vi "TCL Select Fragments 1fragNcriteria.vi"(0 "event file":path, 1 "fragment":string, 3 "primary key":string, 4 "criteria":T1(array[cluster]), 5 "error in (no error)":errorcluster) -> (6 "fragments out":string[](array[string]), 7 "matches":string[][](array[string]), 8 "error out":errorcluster)   [LabVIEW 2010]
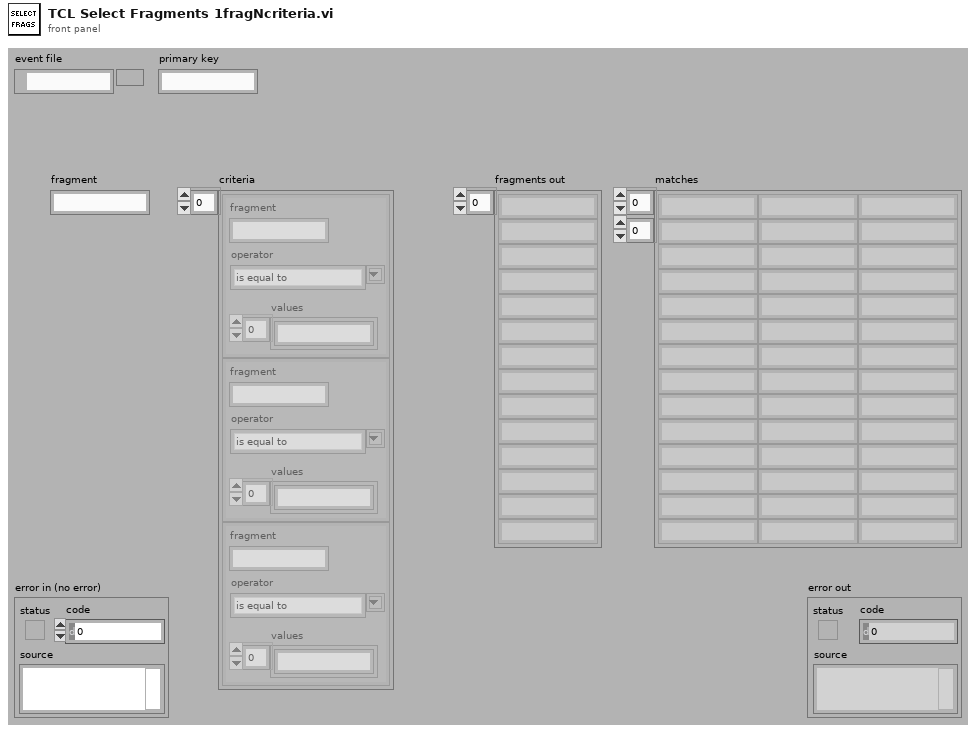
[diagram p1: front panel]
types:
  T1 = cluster{"fragment":string, "values":string[], "operator":string}[]
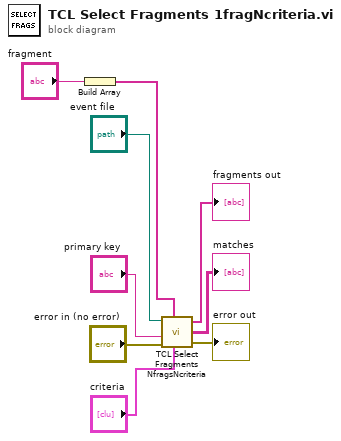
[diagram p0: block diagram]
diagram:
  n1 = Build Array("fragment") -> (w3:string[])
  n2 = call "TCL Select Fragments NfragsNcriteria.vi"("event file"="event file", "fragments"=w3, "primary key"="primary key", "criteria"="criteria", "error in (no error)"="error in (no error)") -> ("fragments out"=→"fragments out":string[], "matches"=→"matches":string[][], "error out"=→"error out":errorcluster)  [unwired: 1 in]
